vi "Write Minimum Level.vi"(10 "Level":T1, 11 "Log Sinks in":refnum<class "Log Sinks.lvclass">) -> (3 "Log Sinks out":refnum<class "Log Sinks.lvclass">)   [LabVIEW 2019, in "TSC Event Logger.lvlib" / "Log Sinks.lvclass"]
uses:
  Log Sinks.lvclass
  Log/Event Level.ctl
  Log Sinks.lvclass/Log Sinks.ctl
  TSC Event Logger.lvlib
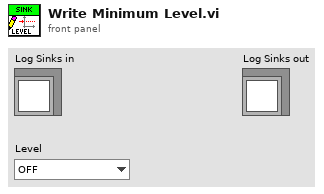
[diagram p1: front panel]
types:
  T1 = typedef "TSC Event Logger.lvlib/Event Level.ctl" = enum16{"OFF", "TRACE", "DEBUG", "INFO", "WARN", "ERROR", "FATAL"}
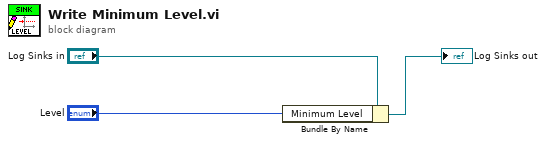
[diagram p0: block diagram]
diagram:
  n1 = Bundle By Name(cluster="Log Sinks in", "Minimum Level"="Level") -> (→"Log Sinks out":refnum<class "Log Sinks.lvclass">)
